vi "Serial_Init.vi"(8 "error in (no error)":errorcluster, 10 "Port":string, 11 "Python":T1) -> (0 "error out":errorcluster, 2 "Console":string, 3 "Python out":T1)   [LabVIEW 2020]
uses:
  PythonCtrl.ctl
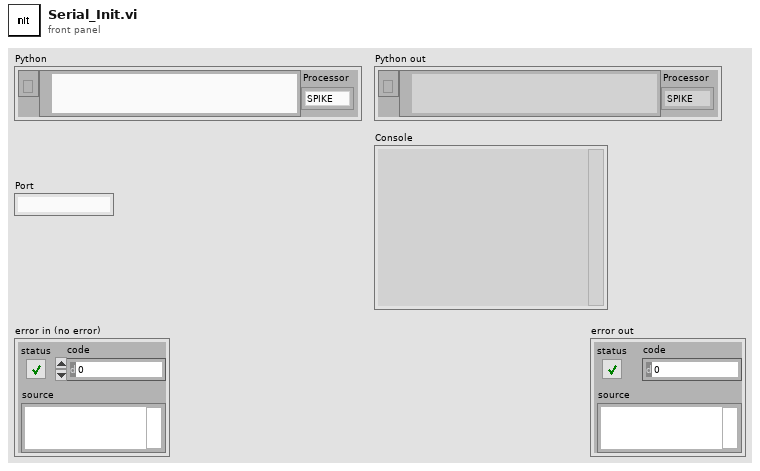
[diagram p1: front panel]
types:
  T1 = typedef "PythonCtrl.ctl" = cluster{"session":refnum<k35>, "PyPath":path, "Processor":enum16{"SPIKE", "Pi"}}
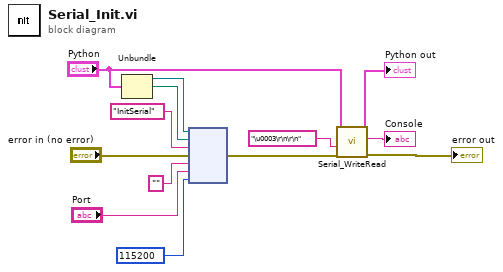
[diagram p0: block diagram]
diagram:
  n1 = Unbundle("Python") -> ("session"=w6:refnum<k35>, "PyPath"=w7:path)  [unwired: 1 out]
  n2 = node(w6, w7, "InitSerial" ("function name"), "error in (no error)", "" ("function name"), "Port", 115200) -> (w2:errorcluster)  [unwired: 3 in, 3 out]
  n3 = call "Serial_WriteRead.vi"("error in (no error)"=w2, "Code"="\u0003\r\n\r\n" ("function name"), "Python"="Python") -> ("error out"=→"error out":errorcluster, "Console"=→"Console":string, "Python"=→"Python out":T1)  [unwired: 6 in]
